vi "Drive_Utils_UpdateState.vi"(6 "error in (no error)":errorcluster, 7 "RobotPosition":cluster{"X":dbl, "Y":dbl, "Angle":dbl}, 8 "speed right":dbl, 9 "speed left":dbl, 10 "delta right":dbl, 11 "delta left":dbl) -> (0 "error out":errorcluster, 2 "deltaPosition":cluster{"X":dbl, "Y":dbl, "Angle":dbl}, 3 "state out":T1)   [LabVIEW 2009, in "Drive.lvlib" / "Drive_Utils.lvlib"]
uses:
  Drive_Utils.lvlib
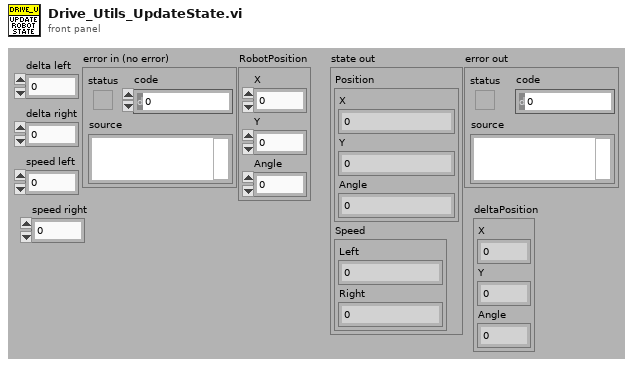
[diagram p1: front panel]
types:
  T1 = cluster{"Position":cluster{"X":dbl, "Y":dbl, "Angle":dbl}, "Speed":cluster{"Left":dbl, "Right":dbl}}
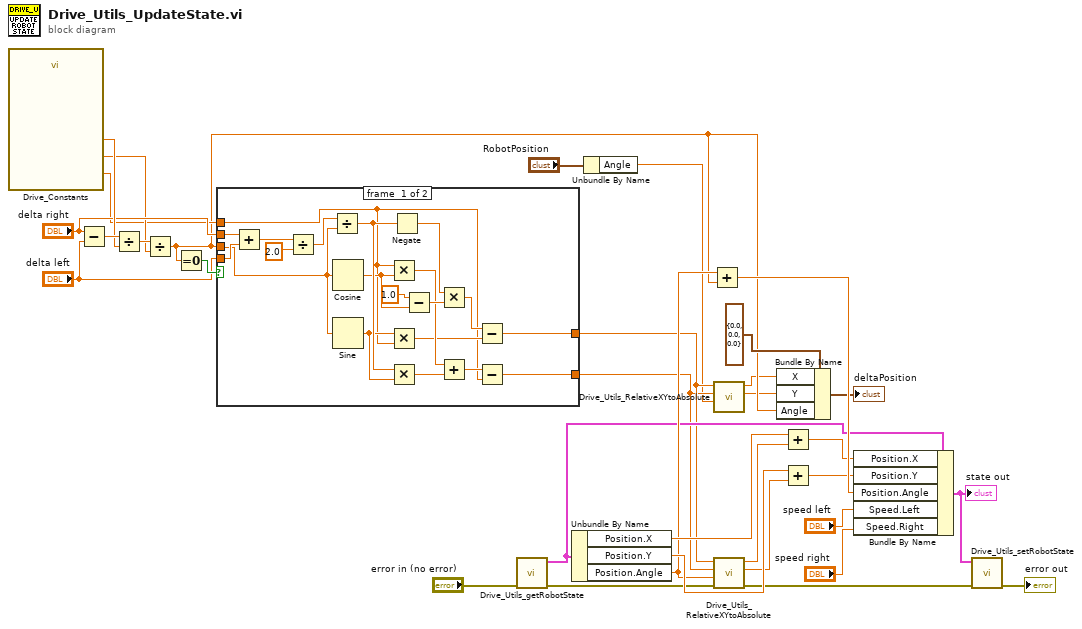
[diagram p0: block diagram]
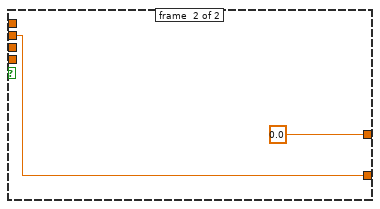
[diagram p2: hidden frame]
diagram:
  n1 = call "Drive_Constants.vi"() -> ("Camera Offset"=w12:dbl, "Wheels interval (m)"=w30:dbl, "Turning correction constant"=w13:dbl)  [unwired: 19 in, 6 out]
  n2 = Subtract(x="delta right", y="delta left") -> (x-y=w31:dbl)
  n3 = Divide(x=w31, y=w30) -> (x/y=w14:dbl)
  n4 = Divide(x=w14, y=w13) -> (x/y=w9:dbl)
  n5 = Equal To 0?(x=w9) -> (x = 0?=w28:bool)
  n6 = case shown="False" w28 {
    tunnel: "delta right" -> [w53 w55]
    tunnel: "delta left" -> [w52 _]
    tunnel: w9 -> [w47 _]
    tunnel: [w42 0.0 ("delta right")] -> w7
    tunnel: [w34 w55] -> w6
    tunnel: w12 -> [w35 _]
    frame #0 {
      n7 = Add(x=w53, y=w52) -> (x+y=w51:dbl)
      n8 = Divide(x=w51, y=2.0) -> (x/y=w49:dbl)
      n9 = Divide(x=w49, y=w47) -> (x/y=w48:dbl)
      n10 = Cosine(x=w47) -> (cos(x)=w40:dbl)
      n11 = Sine(x=w47) -> (sin(x)=w39:dbl)
      n12 = Multiply(x=w35, y=w40) -> (x*y=w41:dbl)
      n13 = Multiply(x=w39, y=w35) -> (x*y=w37:dbl)
      n14 = Multiply(x=w48, y=w39) -> (x*y=w43:dbl)
      n15 = Negate(x=w48) -> (-x=w45:dbl)
      n16 = Subtract(x=1.0, y=w40) -> (x-y=w44:dbl)
      n17 = Multiply(x=w45, y=w44) -> (x*y=w38:dbl)
      n18 = Add(x=w41, y=w43) -> (x+y=w36:dbl)
      n19 = Subtract(x=w38, y=w37) -> (x-y=w42:dbl)
      n20 = Subtract(x=w36, y=w35) -> (x-y=w34:dbl)
    }
    frame #1 {
    }
  }
  n21 = call "Drive_Utils_getRobotState.vi"("error in (no error)"="error in (no error)") -> ("error out"=w18:errorcluster, "Robot State"=w19:T1)  [unwired: 9 in]
  n22 = Unbundle By Name(w19) -> ("Position.X"=w25:dbl, "Position.Y"=w23:dbl, "Position.Angle"=w21:dbl)
  n23 = Unbundle By Name("RobotPosition") -> ("Angle"=w4:dbl)
  n24 = Add(x=w21, y=w9) -> (x+y=w29:dbl)
  n25 = call "Drive_Utils_RelativeXYtoAbsolute.vi"("Angle"=w4, "Y"=w6, "X"=w7) -> ("Y"=w1:dbl, "X"=w2:dbl)  [unwired: 2 in, 1 out]
  n26 = call "Drive_Utils_RelativeXYtoAbsolute.vi"("error in"=w18, "Angle"=w21, "Y"=w6, "X"=w7) -> ("error out"=w16:errorcluster, "Y"=w3:dbl, "X"=w8:dbl)  [unwired: 1 in]
  n27 = Bundle By Name(cluster=cluster{"X":dbl, "Y":dbl, "Angle":dbl} {"X"=0.0, "Y"=0.0, "Angle"=0.0} ("deltaPosition 2"), "X"=w2, "Y"=w1, "Angle"=w9) -> (→"deltaPosition":cluster{"X":dbl, "Y":dbl, "Angle":dbl})
  n28 = Add(x=w25, y=w8) -> (x+y=w24:dbl)
  n29 = Add(x=w23, y=w3) -> (x+y=w22:dbl)
  n30 = Bundle By Name(cluster=w19, "Position.X"=w24, "Position.Y"=w22, "Position.Angle"=w29, "Speed.Left"="speed left", "Speed.Right"="speed right") -> (w17:T1)
  "state out" <- w17
  n31 = call "Drive_Utils_setRobotState.vi"("error in (no error)"=w16, "Robot State"=w17) -> ("error out"=→"error out":errorcluster)  [unwired: 9 in]
